vi "Initialize Tests On Tree.vi"(8 "error in":errorcluster, 9 "Parent Tag (\"\")":string, 10 "tests":refnum<class>[](array[class]), 11 "Tree reference":refnum<vi>) -> (0 "error out":errorcluster, 2 "Tree Methods":i32)   [LabVIEW 2011, in "GraphicalTestRunner.lvlib"]
uses:
  GraphicalTestRunner.lvlib
  Classes/TestSuite/TestSuite.lvclass
  <userlib>/_OpenG.lib/file/file.llb/Strip Path Extension - String__ogtk.vi
  <userlib>/_OpenG.lib/dictionary/dictionary.llb/Dictionary Update (by scalar value)__ogtk.vi
  <userlib>/_OpenG.lib/comparison/comparison.llb/String Changed__ogtk.vi
  Libraries/VITesterUtilities.lvlib
  Classes/TestLoader/TestLoader.lvclass
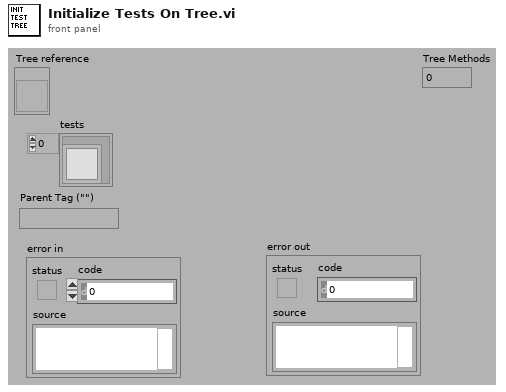
[diagram p1: front panel]
types:
  T1 = typedef "Dictionary Object RefNum__ogtk.ctl" = refnum<k1>
  T2 = cluster{"root":string, "Edit Tree Items:Add Item":string}
  T3 = cluster{"Edit Tree Items:Add Item":string, string[]}
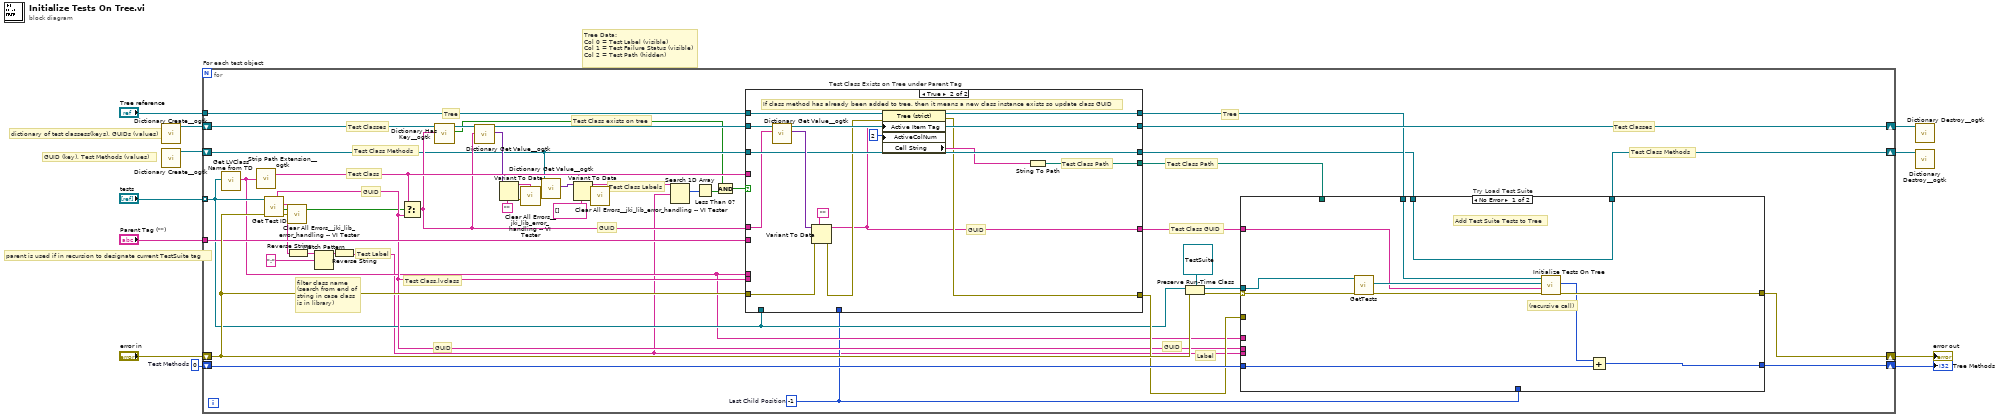
[diagram p0: block diagram]
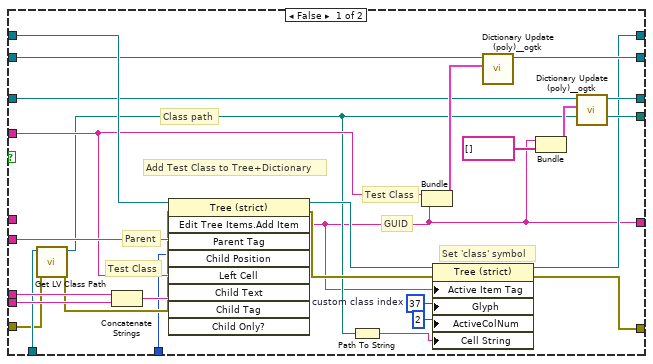
[diagram p2: hidden frame]
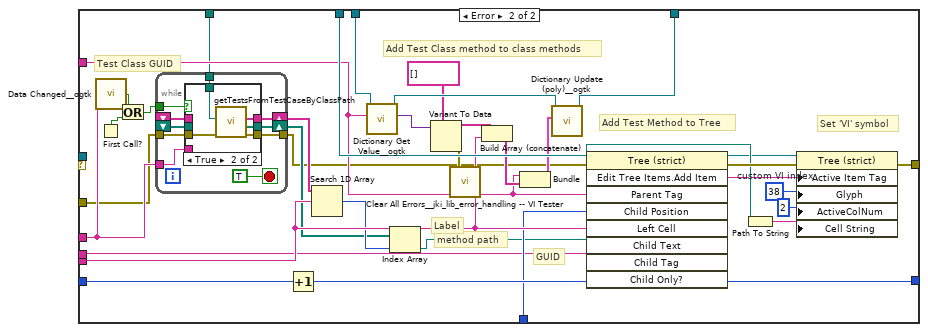
[diagram p3: hidden frame]
diagram:
  w9 = 0  # Test Methods
  # "Tree Data:\nCol 0 = Test Label (visible)\nCol 1 = Test Failure Status (visible)\nCol 2 = Test Path (hidden)"
  # "GUID (key), Test Methods (values)"
  # "dictionary of test classess(keys), GUIDs (values)"
  # "parent is used if in recursion to designate current TestSuite tag"
  n1 = call <userlib>:"Dictionary Create__ogtk.vi"() -> ("dictionary out"=w8:T1)  [unwired: 10 in, 1 out]
  n2 = call <userlib>:"Dictionary Create__ogtk.vi"() -> ("dictionary out"=w6:T1)  [unwired: 10 in, 1 out]
  n3 = for "For each test object" {
    tunnel: "tests" -> [w23] mode=indexing
    shift-right: [w53] -> w2
    shift-left: "error in" -> [w50]
    shift-right: [w51] -> w1
    shift-left: w9 -> [w52]
    tunnel: "Tree reference" -> [w44]
    tunnel: "Parent Tag (\"\")" -> [w46]
    shift-right: [w45] -> w7
    shift-left: w8 -> [w47]
    shift-right: [w25] -> w5
    shift-left: w6 -> [w35]
    w20 = -1  # Last Child Position
    # "Test Class Path"
    # "Test Class Labels"
    # "filter class name\n(search from end of string in case class is in library)"
    # "GUID"
    # "Test Class exists on tree"
    # "Test Class Methods"
    # "Test Classes"
    # "Test Class Methods"
    # "Test Classes"
    # "GUID"
    # "Test Class.lvclass"
    # "GUID"
    # "Label"
    # "Tree"
    # "Tree"
    # "Test Class GUID"
    # "Test Class"
    # "Test Label"
    # "GUID"
    n4 = call "Get LVClass Name from TD.vi"("Variant"=w23) -> ("LVClass Name"=w22:string)  [unwired: 9 in, 1 out]
    n5 = call-poly <userlib>:"Strip Path Extension__ogtk.vi"("path"=w22) -> ("root"=w42:string)  [unwired: 1 out]
    n6 = call "Get Test ID.vi"("error in"=w50, "Test In"=w23) -> ("error out"=w49:errorcluster, "IsTestCase"=w40:bool, "id"=w18:string, "GUID"=w41:string)  [unwired: 5 in, 1 out]
    n7 = call "Clear All Errors__jki_lib_error_handling -- VI Tester.vi"("error in"=w49) -> ()  [unwired: 4 in, 1 out]
    n8 = Reverse String(1:w18) -> (0:w17:string)
    n9 = Match Pattern(string=w17, regular expression=":") -> (before substring=w15:string)  [unwired: 1 in, 3 out]
    n10 = Reverse String(1:w15) -> (0:w16:string)
    n11 = Select(t=w42, s=w40, f=w41) -> (s? t:f=w37:string)
    n12 = call <userlib>:"Dictionary Has Key__ogtk.vi"("key"=w37, "dictionary"=w47) -> ("Has Key?"=w12:bool, "dictionary out"=w14:T1)  [unwired: 7 in, 1 out]
    n13 = call <userlib>:"Dictionary Get Value__ogtk.vi"("key"=w37, "dictionary"=w14) -> ("value"=w38:variant, "dictionary out"=w13:T1)  [unwired: 6 in, 2 out]
    n14 = Variant To Data(type="", Variant=w38) -> (data=w36:string, error out=w27:errorcluster)  [unwired: 1 in]
    n15 = call "Clear All Errors__jki_lib_error_handling -- VI Tester.vi"("error in"=w27) -> ()  [unwired: 4 in, 1 out]
    n16 = call <userlib>:"Dictionary Get Value__ogtk.vi"("key"=w36, "dictionary"=w35) -> ("value"=w33:variant)  [unwired: 6 in, 3 out]
    n17 = Variant To Data(type=string[] [], Variant=w33) -> (data=w32:string[], error out=w28:errorcluster)  [unwired: 1 in]
    n18 = call "Clear All Errors__jki_lib_error_handling -- VI Tester.vi"("error in"=w28) -> ()  [unwired: 4 in, 1 out]
    n19 = Search 1D Array(1D array=w32, element=w16) -> (index of element=w31:i32)  [unwired: 1 in]
    n20 = Less Than 0?(x=w31) -> (x < 0?=w30:bool)
    n21 = Compound Arithmetic op=AND(w12, w30) -> (w29:bool)
    n22 = case "Test Class Exists on Tree under Parent Tag" shown="True" w29 {
      tunnel: w44 -> [w82 w87]
      tunnel: w50 -> [w64 w94]
      tunnel: w46 -> [w81 _]
      tunnel: [w74 w85] -> w48
      tunnel: [w57 w83] -> w24
      tunnel: w13 -> [w80 w97]
      tunnel: w42 -> [w66 _]
      tunnel: [w78 w93] -> w45
      tunnel: w41 -> [w73 _]
      tunnel: [w58 w84] -> w43
      tunnel: w22 -> [w72 _]
      tunnel: w37 -> [_ w91]
      tunnel: w35 -> [w71 w92]
      tunnel: [w70 w92] -> w26
      tunnel: w23 -> [w65 _]
      tunnel: [w60 w88] -> w21
      tunnel: w20 -> [w62 _]
      frame False {
        w77 = 37  # custom class index
        # "Class path"
        # "Set 'class' symbol"
        # "Add Test Class to Tree+Dictionary"
        # "Test Class"
        # "Parent"
        # "Test Class"
        # "GUID"
        n23 = call <vilib>:"Get LV Class Path.vi"("error in (no error)"=w64, "object"=w65) -> ("error out"=w63:errorcluster, "class path"=w60:path)  [unwired: 8 in]
        n24 = Concatenate Strings(w72, w73) -> (w67:string)
        n25 = invoke class="Tree (strict)" method="Edit Tree Items.Add Item"(reference=w82, error in=w63, "Parent Tag"=w81, "Child Position"=w62, "Left Cell"=w66, "Child Tag"=w67) -> (reference out=w76:refnum<vi>, error out=w75:errorcluster, "Edit Tree Items:Add Item"=w57:string)  [unwired: 3 in, 6 out]
        n26 = Path To String(path=w60) -> (string=w59:string)
        n27 = Bundle("root"=w66, "Edit Tree Items:Add Item"=w57) -> (w79:T2)  [unwired: 1 in]
        n28 = property class="Tree (strict)"(reference=w76, error in=w75, "Active Item Tag"=w57, "Glyph"=w77, "ActiveColNum"=2 ("Active Cell:Active Column Number"), "Cell String"=w59) -> (reference out=w58:refnum<vi>, error out=w74:errorcluster)
        n29 = call-poly <userlib>:"Dictionary Update (poly)__ogtk.vi"("key-value"=w79, "dictionary"=w80) -> ("dictionary out"=w78:T1)  [unwired: 7 in, 2 out]
        n30 = Bundle("Edit Tree Items:Add Item"=w57, string[] []) -> (w69:T3)  [unwired: 1 in]
        n31 = call-poly <userlib>:"Dictionary Update (poly)__ogtk.vi"("key-value"=w69, "dictionary"=w71) -> ("dictionary out"=w70:T1)  [unwired: 7 in, 2 out]
      }
      frame True {
        # "If class method has already been added to tree, then it means a new class instance exists so update class GUID"
        # "Test Class Path"
        # "GUID"
        n32 = call <userlib>:"Dictionary Get Value__ogtk.vi"("key"=w91, "dictionary"=w97) -> ("value"=w96:variant, "dictionary out"=w93:T1)  [unwired: 6 in, 2 out]
        n33 = Variant To Data(error in=w94, type="", Variant=w96) -> (data=w83:string, error out=w86:errorcluster)
        n34 = property class="Tree (strict)"(reference=w87, error in=w86, "Active Item Tag"=w83, "ActiveColNum"=2 ("Active Cell:Active Column Number")) -> (reference out=w84:refnum<vi>, error out=w85:errorcluster, "Cell String"=w89:string)
        n35 = String To Path(string=w89) -> (path=w88:path)
      }
    }
    n36 = Preserve Run-Time Class(object in=w23, error in=w50, 2:refnum<class "TestSuite.lvclass"> refnum ("TestSuite.lvclass")) -> (object out=w54:refnum<class "TestSuite.lvclass">, error out=w55:errorcluster)
    n37 = case "Try Load Test Suite" shown="No Error" w55 {
      selector: w55 -> [w100 _]
      tunnel: w54 -> [w108 _]
      tunnel: [w105 w137] -> w53
      tunnel: w52 -> [w102 w142]
      tunnel: [w104 w141] -> w51
      tunnel: w43 -> [w99 w140]
      tunnel: w48 -> [_ w119]
      tunnel: w24 -> [w98 w131]
      tunnel: w16 -> [_ w125]
      tunnel: w41 -> [_ w110]
      tunnel: w26 -> [w101 w136]
      tunnel: [w101 w128] -> w25
      tunnel: w22 -> [_ w122]
      tunnel: w21 -> [_ w116]
      tunnel: w20 -> [_ w115]
      frame No Error {
        # "(recursive call)"
        # "Add Test Suite Tests to Tree"
        n38 = call-dynamic "GetTests.vi"("error in (no error)"=w100, "TestSuite in"=w108) -> ("error out"=w106:errorcluster, "tests"=w107:refnum<class>[])  [unwired: 7 in, 1 out]
        n39 = call "Initialize Tests On Tree.vi"("error in"=w106, "Parent Tag (\"\")"=w98, "tests"=w107, "Tree reference"=w99) -> ("error out"=w105:errorcluster, "Tree Methods"=w103:i32)  [unwired: 6 in]
        n40 = Add(x=w103, y=w102) -> (x+y=w104:i32)
      }
      frame Error {
        w139 = 38  # custom VI index
        # "method path"
        # "Add Test Class method to class methods"
        # "Test Class GUID"
        # "Label"
        # "GUID"
        # "Set 'VI' symbol"
        # "Add Test Method to Tree"
        n41 = call-poly <userlib>:"Data Changed__ogtk.vi"("String"=w122) -> ("Changed"=w121:bool)
        n42 = First Call?() -> (First Call?: T/F=w120:bool)
        n43 = Or(x=w121, y=w120) -> (x .or. y?=w117:bool)
        n44 = while {
          tunnel: w122 -> [w150]
          tunnel: w119 -> [w149]
          tunnel: [w148] -> w118
          shift-right: [w152] -> w126
          shift-left: _ -> [w145]
          shift-right: [w151] -> w123
          shift-left: _ -> [w144]
          tunnel: w117 -> [w146]
          tunnel: w116 -> [w143]
          stop <- TRUE stop-if-true
          n45 = case shown="True" w146 {
            tunnel: [w154 w160] -> w152
            tunnel: [w153 w159] -> w151
            tunnel: w150 -> [_ _]
            tunnel: w149 -> [w155 w156]
            tunnel: [w155 w158] -> w148
            tunnel: w145 -> [w154 _]
            tunnel: w144 -> [w153 _]
            tunnel: w143 -> [_ w157]
            frame False {
            }
            frame True {
              n46 = call "getTestsFromTestCaseByClassPath.vi"("error in"=w156, "TestCase Path"=w157) -> ("error out"=w158:errorcluster, "test paths"=w159:path[], "tests"=w160:string[])  [unwired: 7 in]
            }
          }
        }
        n47 = Increment(x=w142) -> (x+1=w141:i32)
        n48 = Search 1D Array(1D array=w126, element=w125) -> (index of element=w124:i32)  [unwired: 1 in]
        n49 = call <userlib>:"Dictionary Get Value__ogtk.vi"("key"=w131, "dictionary"=w136) -> ("value"=w134:variant, "dictionary out"=w135:T1)  [unwired: 6 in, 2 out]
        n50 = Index Array(array=w123, index=w124) -> (element=w113:path)
        n51 = Variant To Data(type=string[] [], Variant=w134) -> (data=w133:string[], error out=w129:errorcluster)  [unwired: 1 in]
        n52 = call "Clear All Errors__jki_lib_error_handling -- VI Tester.vi"("error in"=w129) -> ()  [unwired: 4 in, 1 out]
        n53 = Build Array (concatenate)(w133, w125) -> (w132:string[])
        n54 = Bundle("Edit Tree Items:Add Item"=w131, w132) -> (w130:T3)  [unwired: 1 in]
        n55 = call-poly <userlib>:"Dictionary Update (poly)__ogtk.vi"("key-value"=w130, "dictionary"=w135) -> ("dictionary out"=w128:T1)  [unwired: 7 in, 2 out]
        n56 = invoke class="Tree (strict)" method="Edit Tree Items.Add Item"(reference=w140, error in=w118, "Parent Tag"=w131, "Child Position"=w115, "Left Cell"=w125, "Child Tag"=w110) -> (reference out=w109:refnum<vi>, error out=w138:errorcluster, "Edit Tree Items:Add Item"=w111:string)  [unwired: 3 in, 6 out]
        n57 = Path To String(path=w113) -> (string=w112:string)
        n58 = property class="Tree (strict)"(reference=w109, error in=w138, "Active Item Tag"=w111, "Glyph"=w139, "ActiveColNum"=2 ("Active Cell:Active Column Number"), "Cell String"=w112) -> (error out=w137:errorcluster)  [unwired: 1 out]
      }
    }
  }
  "error out" <- w2
  "Tree Methods" <- w1
  n59 = call <userlib>:"Dictionary Destroy__ogtk.vi"("dictionary"=w7) -> ()  [unwired: 10 in, 1 out]
  n60 = call <userlib>:"Dictionary Destroy__ogtk.vi"("dictionary"=w5) -> ()  [unwired: 10 in, 1 out]
